vi "Unflatten.vi"(8 "error in (no error)":errorcluster, 11 "Translation Stage in":refnum<class "Translation Stage.lvclass">) -> (0 "error out":errorcluster, 3 "Translation Stage out":refnum<class "Translation Stage.lvclass">)   [LabVIEW 2009, in "Translation Stage.lvclass"]
uses:
  Translation Stage.lvclass
  Scanner/Scanner.lvclass
  Global/File Locations.vi
  Translation Stage.lvclass/Translation Stage.ctl
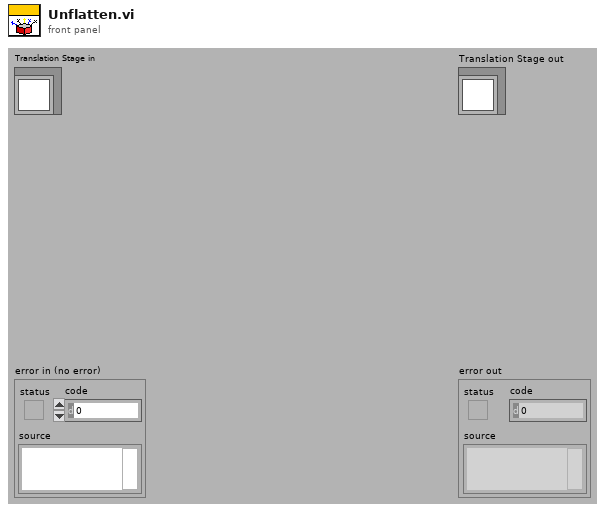
[diagram p1: front panel]
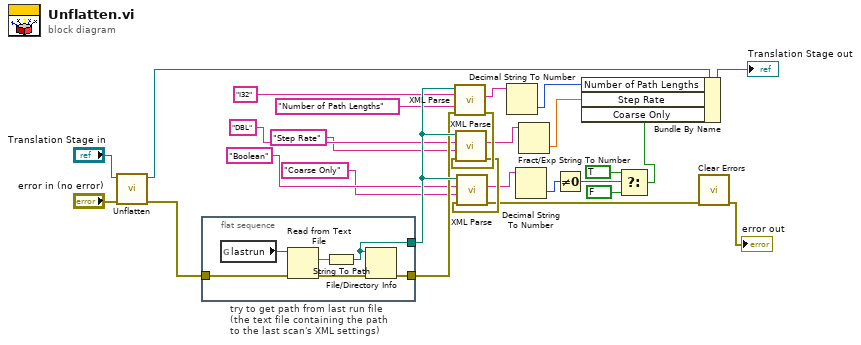
[diagram p0: block diagram]
diagram:
  n1 = call-parent "Unflatten.vi"("error in (no error)"="error in (no error)", "Scanner in"="Translation Stage in") -> ("error out"=w23:errorcluster, "Scanner out"=w27:refnum<class "Translation Stage.lvclass">)  [unwired: 8 in]
  n2 = flat-sequence "try to get path from last run file\n(the text file containing the path\nto the last scan's XML settings)" {
    tunnel: [w33] -> w22
    tunnel: [w29] -> w21
    tunnel: w23 -> [w28]
    frame #0 {
      n3 = global read "File Locations.vi" "lastrun"() -> (w31:path)
      n4 = Read from Text File(file (use dialog)=w31, error in=w28) -> (text=w32:string, error out=w30:errorcluster)  [unwired: 4 out]
      n5 = String To Path(string=w32) -> (path=w33:path)
      n6 = File/Directory Info(path=w33, error in=w30) -> (error out=w29:errorcluster)  [unwired: 6 out]
    }
  }
  n7 = call "XML Parse.vi"("error in (no error)"=w21, "Name String"="Number of Path Lengths", "Type String"="I32", "Path"=w22) -> ("error out"=w20:errorcluster, "String Out"=w12:string)  [unwired: 6 in]
  n8 = call "XML Parse.vi"("error in (no error)"=w20, "Name String"="Step Rate", "Type String"="DBL", "Path"=w22) -> ("error out"=w19:errorcluster, "String Out"=w10:string)  [unwired: 6 in]
  n9 = call "XML Parse.vi"("error in (no error)"=w19, "Name String"="Coarse Only", "Type String"="Boolean", "Path"=w22) -> ("error out"=w8:errorcluster, "String Out"=w7:string)  [unwired: 6 in]
  n10 = Decimal String To Number(string=w12) -> (number=w11:i32)  [unwired: 2 in, 1 out]
  n11 = Decimal String To Number(string=w7) -> (number=w4:i32)  [unwired: 2 in, 1 out]
  n12 = Fract/Exp String To Number(string=w10) -> (number=w9:dbl)  [unwired: 3 in, 1 out]
  n13 = Not Equal To 0?(x=w4) -> (x != 0?=w3:bool)
  n14 = Select(t=TRUE, s=w3, f=FALSE) -> (s? t:f=w2:bool)
  n15 = Bundle By Name(cluster=w27, "Number of Path Lengths"=w11, "Step Rate"=w9, "Coarse Only"=w2) -> (→"Translation Stage out":refnum<class "Translation Stage.lvclass">)
  n16 = call <vilib>:"Clear Errors.vi"("error in (no error)"=w8) -> ("error out"=→"error out":errorcluster)  [unwired: 6 in]
